vi "FGV.vi"(7 "Mode":T1=enum."Read", 8 "error in":errorcluster, 10 "Board Pins In":T2[](array[typedef]) {"Index"."DigitalIndex" step=1 format="D%d"; "Index"."AnalogIndex" min=0.0 step=1.0 format="A%#.0g"}, 11 "comport":refnum<visa-resource-name>) -> (0 "error out":errorcluster, 2 "Board Pins Out":T2[](array[typedef]) {"Index"."DigitalIndex" step=1 format="D%d"; "Index"."AnalogIndex" min=0.0 step=1.0 format="A%#.0g"}, 3 "comport out":refnum<visa-resource-name>)   [LabVIEW 2020, in "FirmataClient.lvlib"]
doc: "FGV to be used to store uut's io states for asynchronous consumption"
uses:
  FirmataClient.lvlib
  controls/FGV-Mode.ctl
  controls/PinModesListData.ctl
  controls/PinModeData.ctl
  controls/FirmataPinModes.ctl
  controls/BoardPinsCapabilities.ctl
panel:
  out "Firmata Modes":string[](array[string])
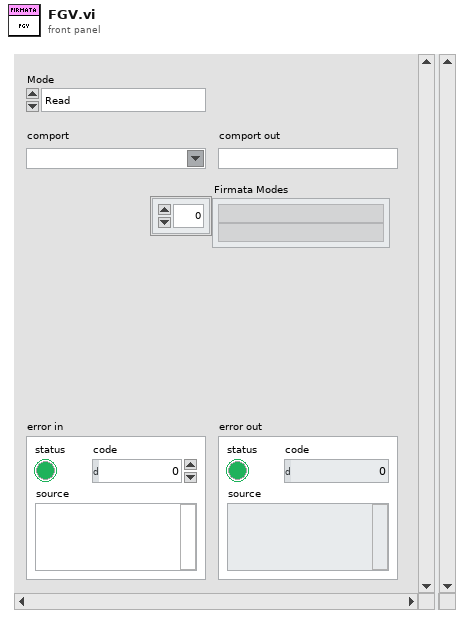
[diagram p1: front panel]
types:
  T1 = typedef "FirmataClient.lvlib/FGV-Mode.ctl" = enum16{"Load Comport", "Load Board Capabilities", "Read"}
  T2 = typedef "FirmataClient.lvlib/PinModesListData.ctl" = cluster{"DigitalInputMode":T3, "DigitalOutputMode":T3, "AnalogInputMode":T3, "PWMMode":T3, "ServoMode":T3, "ShiftMode":T3, "I2CMode":T3, "OneWireMode":T3, "StepperMode":T3, "EncoderMode":T3, "SerialMode":T3, "InputPullupMode":T3, "Ext.SPIMode":T3, "Ext.SonarMode":T3, "Ext.ToneMode":T3, "Ext.DHTMode":T3, "Index":cluster{"DigitalIndex":u16, "AnalogIndex":dbl}}
  T3 = typedef "FirmataClient.lvlib/PinModeData.ctl" = cluster{"Resolution":u8, "btn":bool, "PinMode":T4}
  T4 = typedef "FirmataClient.lvlib/FirmataPinModes.ctl" = enum16{"DigitalInput", "DigitalOutput", "AnalogInput", "PWM", "Servo", "Shift", "I2C", "OneWire", "Stepper", "Encoder", "Serial", "InputPullup", "Extended.SPI", "Extended.Sonar", "Extended.Tone", "Extended.DHT"}
  T5 = typedef "FirmataClient.lvlib/BoardPinsCapabilities.ctl" = cluster{"comport":refnum<visa-resource-name>, "Board Pins":T2[]}
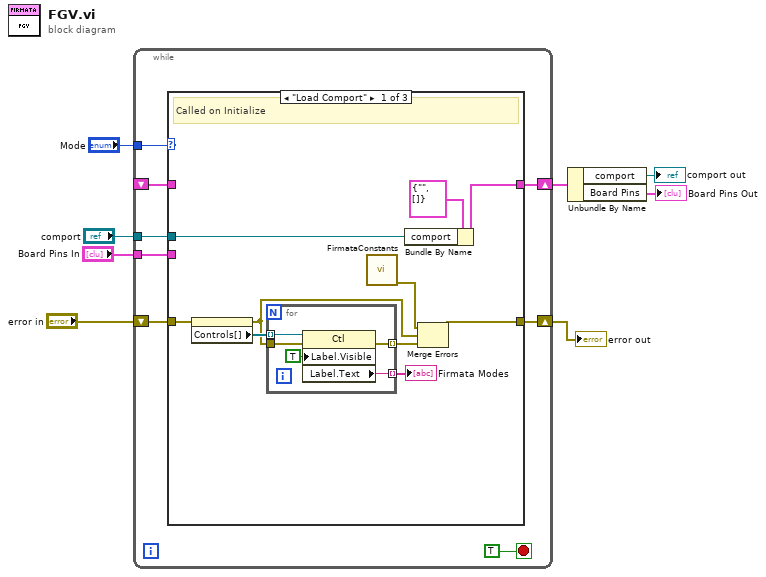
[diagram p0: block diagram]
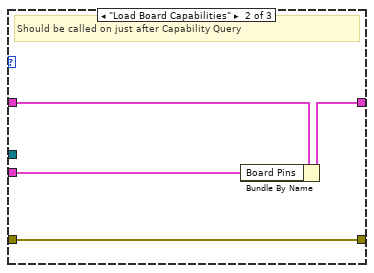
[diagram p2: hidden frame]
diagram:
  n1 = while {
    tunnel: "Mode" -> [w16]
    shift-right: [w13] -> w6
    shift-left: _ -> [w14]
    tunnel: "comport" -> [w12]
    tunnel: "Board Pins In" -> [w11]
    shift-right: [w10] -> w2
    shift-left: "error in" -> [w9]
    stop <- TRUE stop-if-true
    n2 = case shown="\"Load Comport\"" w16 {
      tunnel: w14 -> [_ w34 w37]
      tunnel: [w25 w35 w37] -> w13
      tunnel: w12 -> [w26 _ _]
      tunnel: w11 -> [_ w33 _]
      tunnel: w9 -> [w21 w32 w36]
      tunnel: [w19 w32 w36] -> w10
      frame "Load Comport" {
        # "Called on Initialize"
        n3 = property class="Clust (strict)"(error in=w21) -> (error out=w18:errorcluster, "Controls[]"=w23:refnum<vi>[])  [unwired: 1 in, 1 out]
        n4 = for {
          tunnel: w23 -> [w31] mode=indexing
          tunnel: [w29] -> w22 mode=indexing
          tunnel: w18 -> [w28]
          tunnel: [w27] -> w20 mode=indexing
          n5 = property on="Property Node" class="Ctl"(reference=w31, error in=w28, "Label.Visible"=TRUE) -> (error out=w27:errorcluster, "Label.Text"=w29:string)  [unwired: 1 out]
        }
        "Firmata Modes" <- w22
        n6 = call "FirmataConstants.vi"() -> ("error out"=w17:errorcluster)  [unwired: 10 in, 1 out]
        n7 = Bundle By Name(cluster=T5 {"comport"="", "Board Pins"=[]}, "comport"=w26) -> (w25:T5)
        n8 = Merge Errors(w17, w18, w20) -> (w19:errorcluster)
      }
      frame "Load Board Capabilities" {
        # "Should be called on just after Capability Query"
        n9 = Bundle By Name(cluster=w34, "Board Pins"=w33) -> (w35:T5)
      }
      frame Default {
      }
    }
  }
  "error out" <- w2
  n10 = Unbundle By Name(w6) -> ("comport"=→"comport out":refnum<visa-resource-name>, "Board Pins"=→"Board Pins Out":T2[])
